vi "check_range.vi"(5 "Attribute Value":dbl, 7 "Attribute":T2={"Identifier"="", "Descriptive name"="", "Data Type"=enum."Integer 32", "Command"="", "Access"=2, "Range Table"="", "Read Callback"="", "Write Callback"="", "Range Callback"="", "Check Callback"="", "Rngtable Callback"="", "Coerce Callback"="", "Supported Models"="", "Instrument Options"="", "Repeated Capabilities"="", "Check Status Callback"="", "Index"=0, "Flag: OPC Wait"=FALSE, "Flag: Dont check status"=FALSE, "Flag: Cache Only"=FALSE} {"Access" items=["Read Only", "Write Only", "Read/Write"]}, 8 "error in":errorcluster, 10 "Mode (Check range from Session)":T1(ring)=enum."Check range from Session", 11 "VISA resource name":refnum<visa-resource-name>) -> (0 "error out":errorcluster, 1 "Enum output":string, 2 "Enum?":bool, 3 "VISA resource name out":refnum<visa-resource-name>)   [LabVIEW 2014, in "rszvl_rsidr_core.lvlib"]
uses:
  rszvl_rsidr_core.lvlib
  type_Attribute.ctl
  type_Attribute_Data_Type.ctl
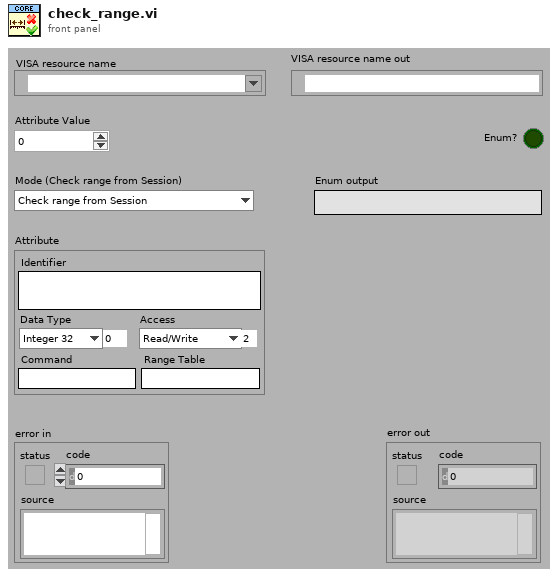
[diagram p1: front panel]
types:
  T1 = enum16{"Check range", "Don't check range", "Check range from Session"}
  T2 = typedef "rszvl_rsidr_core.lvlib/type_Attribute.ctl" = cluster{"Identifier":string, "Descriptive name":string, "Data Type":T3, "Command":string, "Access":u16, "Range Table":string, "Read Callback":string, "Write Callback":string, "Range Callback":string, "Check Callback":string, "Rngtable Callback":string, "Coerce Callback":string, "Supported Models":string, "Instrument Options":string, "Repeated Capabilities":string, "Check Status Callback":string, "Index":i32, "Flag: OPC Wait":bool, "Flag: Dont check status":bool, "Flag: Cache Only":bool}
  T3 = typedef "rszvl_rsidr_core.lvlib/type_Attribute_Data_Type.ctl" = enum16{"Integer 32", "Double", "String", "Boolean", "None", "Integer 64"}
  T4 = enum16{"Initialize", "Check", "Get Numeric Value", "Get Default Value"}
  T5 = typedef "rszvl_rsidr_core.lvlib/type_Session_Data.ctl" = cluster{"Instr type":string, "Instr type for err. msg.":string, "Installed Options":string[], "OPC Timeout":i32, "Query Instrument Status":bool, "Check Range":bool, "Check Options":bool, "Add LF to Write":bool, "Simulate":bool, "Logging":bool, "Logging params":variant, "Interface Type":enum16{"Unknown", "GPIB", "VXI", "GPIB_VXI", "ASRL", "PXI", "TCPIP", "USB", "SOCKET"}, "Fast Sweep":i32, "AdditionalFlags":i32, "WaitBeforeWrite":i32, "WaitBeforeRead":i32, "BinDataChunkSize":i64}
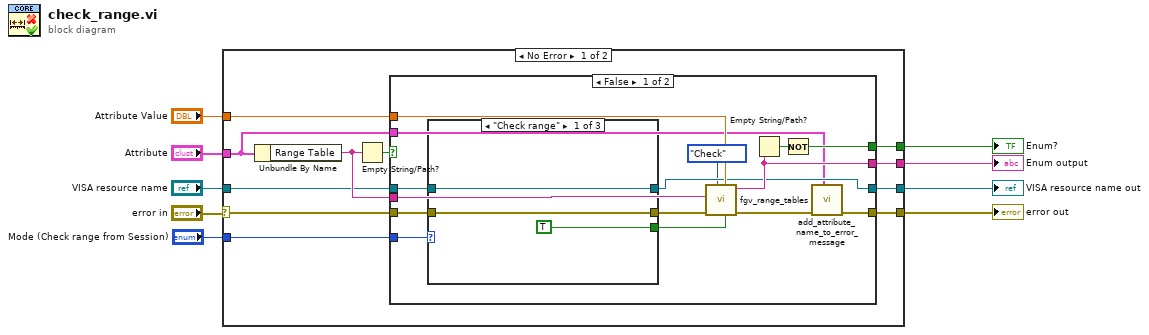
[diagram p0: block diagram]
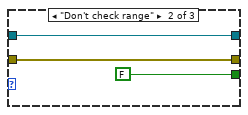
[diagram p2: hidden frame]
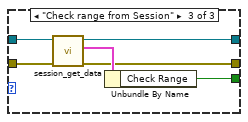
[diagram p3: hidden frame]
diagram:
  n1 = case shown="No Error" "error in" {
    selector: "error in" -> [w15 w51]
    tunnel: [w19 w51] -> w9
    tunnel: "VISA resource name" -> [w16 w50]
    tunnel: [w17 w50] -> w6
    tunnel: "Attribute" -> [w11 _]
    tunnel: [w14 _] -> w4
    tunnel: "Attribute Value" -> [w13 _]
    tunnel: [w12 _] -> w2
    tunnel: "Mode (Check range from Session)" -> [w10 _]
    frame No Error {
      n2 = Unbundle By Name(w11) -> ("Range Table"=w18:string)
      n3 = Empty String/Path?(string/path=w18) -> (empty?=w20:bool)
      n4 = case shown="False" w20 {
        tunnel: w15 -> [w30 w49]
        tunnel: [w24 w49] -> w19
        tunnel: w18 -> [w31 _]
        tunnel: w16 -> [w29 w48]
        tunnel: [w28 w48] -> w17
        tunnel: [w33 _] -> w14
        tunnel: w13 -> [w35 _]
        tunnel: [w32 _] -> w12
        tunnel: w11 -> [w23 _]
        tunnel: w10 -> [w25 _]
        frame False {
          n5 = case shown="\"Check range\"" w25 {
            tunnel: w29 -> [w38 w41 w47]
            tunnel: [w38 w41 w46] -> w28
            tunnel: [w36 w39 w42] -> w26
            tunnel: [TRUE ("Boolean Out") FALSE ("Boolean Out") w45] -> w27
            tunnel: w30 -> [w36 w39 w43]
            frame "Check range" {
            }
            frame "Don't check range" {
            }
            frame "Check range from Session" {
              n6 = call "session_get_data.vi"("error in"=w43, "VISA resource name"=w47) -> ("error out"=w42:errorcluster, "Session User Data out"=w44:T5, "VISA resource name out"=w46:refnum<visa-resource-name>)  [unwired: 7 in]
              n7 = Unbundle By Name(w44) -> ("Check Range"=w45:bool)
            }
          }
          n8 = call "fgv_range_tables.vi"("Range Checking"=w27, "Attribute Value in (0.0)"=w35, "Operation"=T4."Check", "error in"=w26, "Range Table ID in"=w31) -> ("error out"=w22:errorcluster, "Enum output"=w32:string)  [unwired: 3 in, 2 out]
          n9 = Empty String/Path?(string/path=w32) -> (empty?=w34:bool)
          n10 = Not(x=w34) -> (.not. x?=w33:bool)
          n11 = call "add_attribute_name_to_error_message.vi"("Attribute"=w23, "error in"=w22) -> ("error out"=w24:errorcluster)  [unwired: 8 in, 1 out]
        }
        frame True {
        }
      }
    }
    frame Error {
    }
  }
  "VISA resource name out" <- w6
  "error out" <- w9
  "Enum?" <- w4
  "Enum output" <- w2
